vi "Integration Reset.vi"(8 "error in (no error)":errorcluster, 10 "Card #":u8, 11 "Yokogawa WT1600 in":refnum<class "Yokogawa WT1600.lvclass">) -> (0 "error out":errorcluster, 2 "VISA resource name":refnum<visa-resource-name>, 3 "Yokogawa WT1600 out":refnum<class "Yokogawa WT1600.lvclass">)   [LabVIEW 2013, in "Universal Power Meter.lvlib" / "Yokogawa WT1600.lvlib" / "Yokogawa WT1600.lvclass"]
uses:
  Yokogawa WT1600.lvclass
  Universal Power Meter class/Universal Power Meter.lvclass
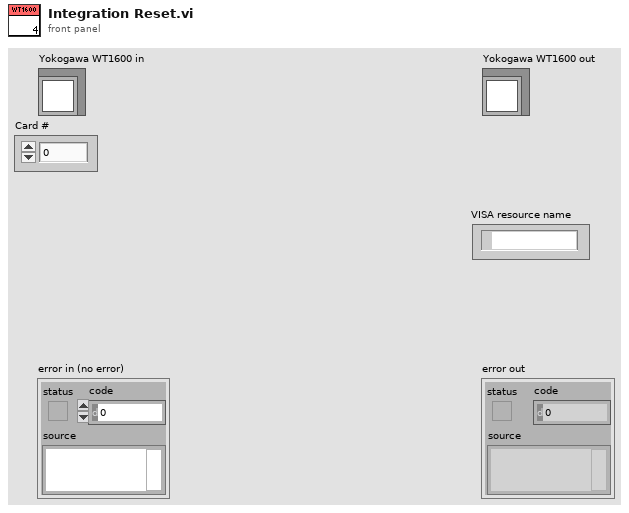
[diagram p1: front panel]
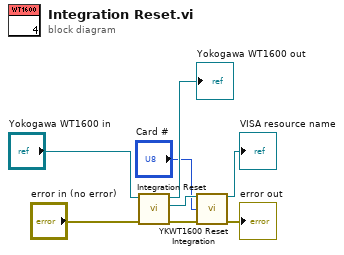
[diagram p0: block diagram]
diagram:
  n1 = call-parent "Integration Reset.vi"("error in (no error)"="error in (no error)", "Universal Power Meter in"="Yokogawa WT1600 in") -> ("error out"=w3:errorcluster, "VISA resource name"=w2:refnum<visa-resource-name>, "Universal Power Meter out"=→"Yokogawa WT1600 out":refnum<class "Yokogawa WT1600.lvclass">)  [unwired: 7 in]
  n2 = call <instrlib>:"YKWT1600 Reset Integration.vi"("VISA session"=w2, "Element (All: 0)"="Card #", "error in (no error)"=w3) -> ("dup VISA session"=→"VISA resource name":refnum<visa-resource-name>, "error out"=→"error out":errorcluster)  [unwired: 11 in]
